vi "proj 2.vi"() -> ()   [LabVIEW 2022 SP3]
panel:
  out "Output":dbl
  out "Previous Iteration":dbl
  out "Top Iteration":dbl
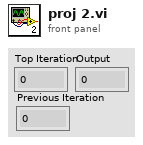
[diagram p1: front panel]
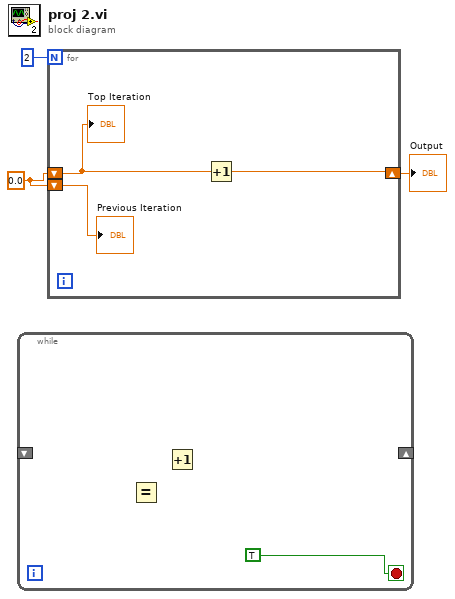
[diagram p0: block diagram]
diagram:
  w3 = 0.0
  n1 = while {
    shift-right: _ -> [_]
    shift-left: _ -> [_]
    stop <- TRUE stop-if-true
    n2 = Equal?() -> ()  [unwired: 2 in, 1 out]
    n3 = Increment() -> ()  [unwired: 1 in, 1 out]
  }
  n4 = for {
    N: 2 -> [_]
    shift-right: [w5] -> w2
    shift-left: w3 -> [w7]
    shift-left: w3 -> [w6]
    n5 = Increment(x=w6) -> (x+1=w5:dbl)
    "Top Iteration" <- w6
    "Previous Iteration" <- w7
  }
  "Output" <- w2
